vi "exersise 3-8.vi"() -> ()   [LabVIEW 2014]
panel:
  out "warning 2":bool
  out "warning text 2":string
  in  "Min Temp 2":dbl
  in  "Max Temp":dbl
  in  "Current Temp":dbl
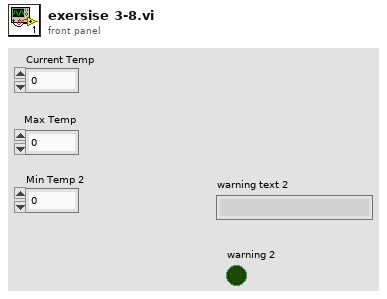
[diagram p1: front panel]
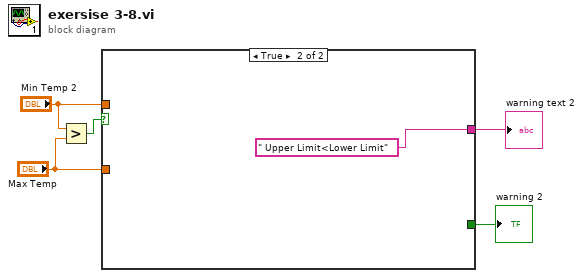
[diagram p0: block diagram]
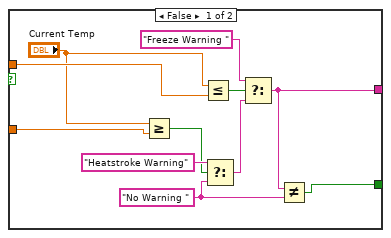
[diagram p2: hidden frame]
diagram:
  n1 = Greater?(x="Min Temp 2", y="Max Temp") -> (0:w5:bool)
  n2 = case shown="True" w5 {
    tunnel: "Max Temp" -> [w10 _]
    tunnel: "Min Temp 2" -> [w9 _]
    tunnel: [w7 " Upper Limit<Lower Limit"] -> w2
    tunnel: [w6 _] -> w1
    frame False {
      w13 = "No Warning "
      n3 = Greater Or Equal?(x="Current Temp", y=w10) -> (x >= y?=w11:bool)
      n4 = Less Or Equal?(x="Current Temp", y=w9) -> (x <= y?=w12:bool)
      n5 = Select(t="Heatstroke Warning", s=w11, f=w13) -> (s? t:f=w15:string)
      n6 = Select(t="Freeze Warning ", s=w12, f=w15) -> (s? t:f=w7:string)
      n7 = Not Equal?(x=w7, y=w13) -> (x != y?=w6:bool)
    }
    frame True {
    }
  }
  "warning 2" <- w1
  "warning text 2" <- w2
